vi "Periodic Tasks.vi"(8 "error in":errorcluster) -> ()   [LabVIEW 2016]
doc: "This VI runs in parallel to other tasks. It can contain as many user-defined periodic loops as you need. These can carry out PID or other sorts of timed response."
uses:
  MotionProfileClass/MotionProfiles.lvclass
  <vilib>/Rock Robotics/WPI/ThirdParty/CanMotor/TalonSRX/WPI_CANTalonSRX_APIControlMode.ctl
  <vilib>/Rock Robotics/WPI/Utilities/WPI_GetSetVariantRefNum.vi
panel:
  out "Left Prof Count":i32
  out "Right Prof Count":i32
  out "Right Throttle":dbl(graph)
  out "Right Motor":T1(graph)
  out "Left Throttle":dbl(graph)
  out "Left Motor":T1(graph)
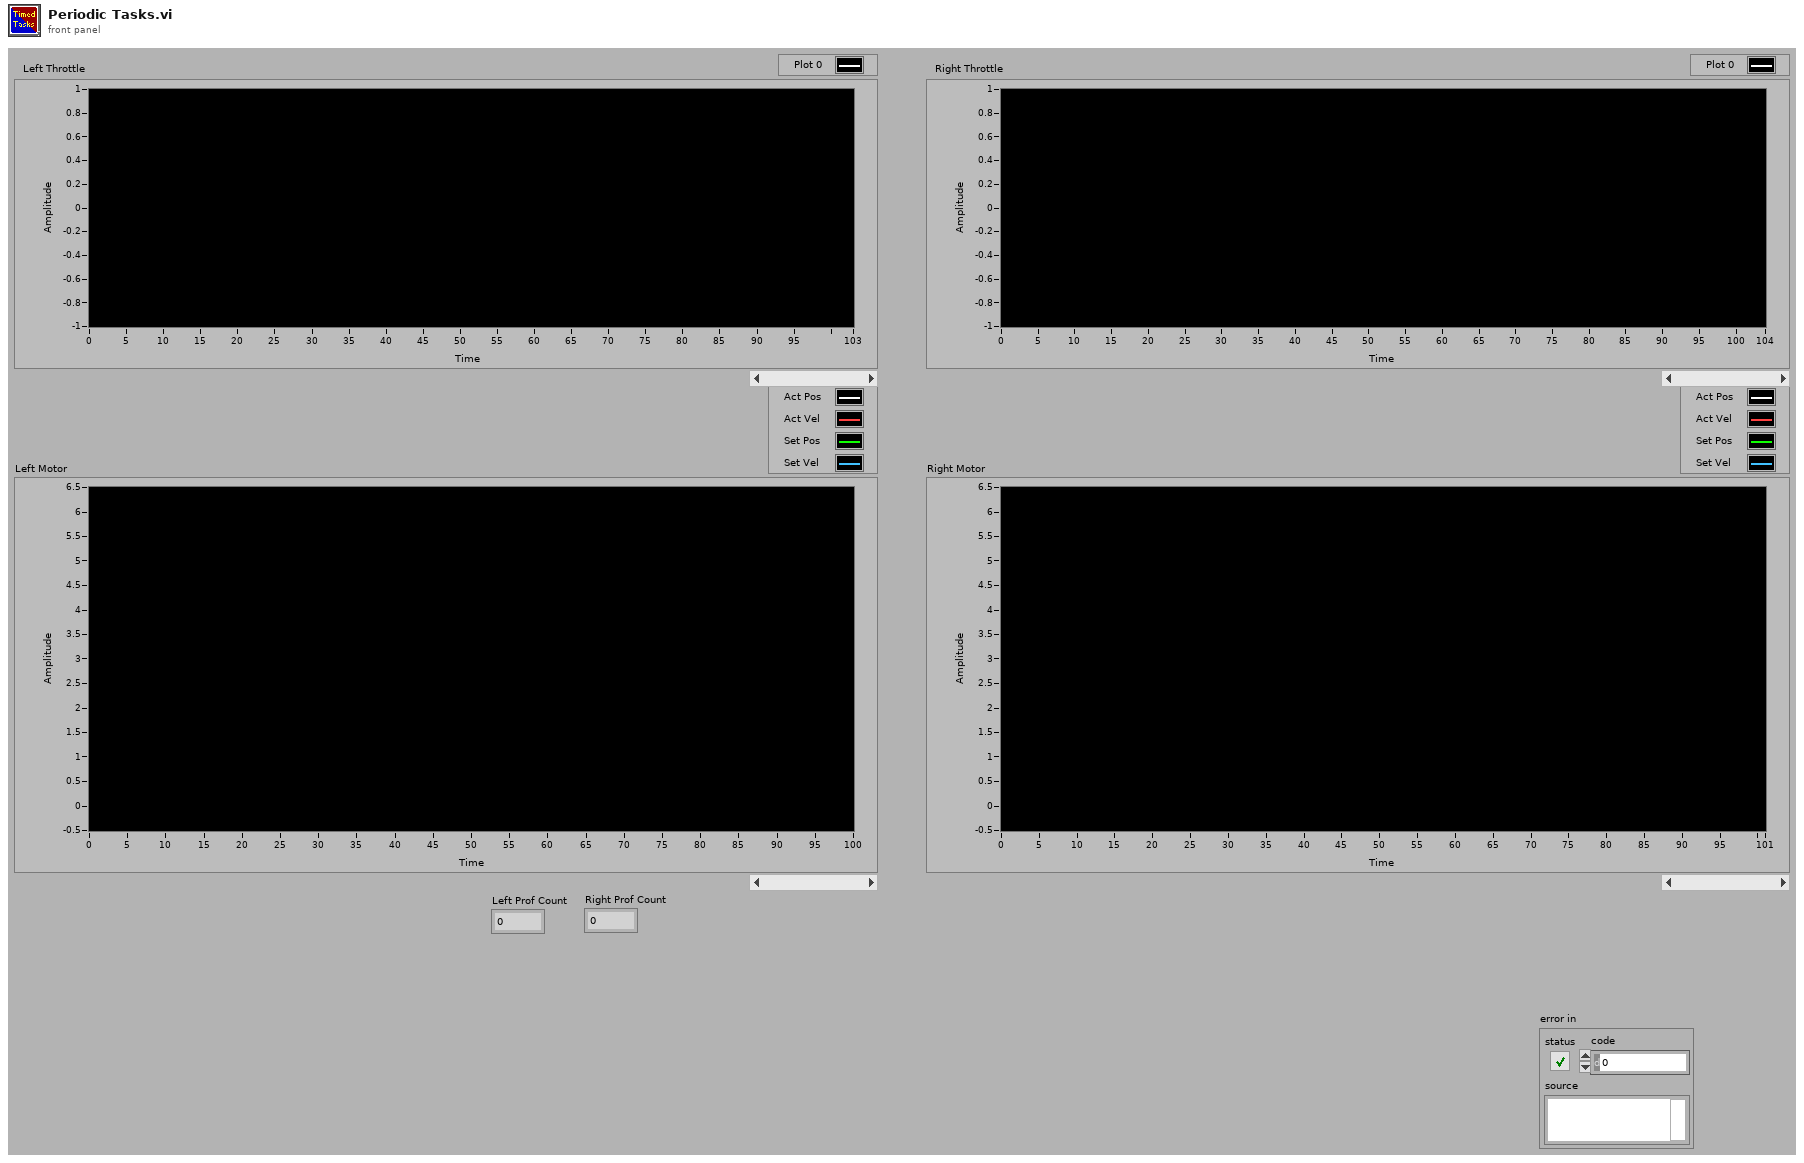
[diagram p1: front panel]
types:
  T1 = cluster{"Sensor Position":dbl, "Sensor Velocity":dbl, "Mot Prof Active Position":dbl, "Mot Prof Active Velocity":dbl}
  T2 = typedef "WPI_MotorControlDeviceRef.ctl" = cluster{"DeviceStatus":errorcluster, "Type":T3, "PWM":cluster{"PWM Channel":T4, "DeadBand":T5}, "CAN":cluster{"Device Number":u8, "SetOutput VI Ref":variant, "GetOutput VI Ref":variant, "Enable VI Ref":variant, "Disable VI Ref":variant, "Data":variant}, "Invert":bool}
  T3 = typedef "WPI_MotorControlType.ctl" = enum16{"PWM", "CAN"}
  T4 = typedef "FPGA_DIOPWMChannel.ctl" = enum8{"PWM 0", "PWM 1", "PWM 2", "PWM 3", "PWM 4", "PWM 5", "PWM 6", "PWM 7", "PWM 8", "PWM 9", "PWM MXP 0", "PWM MXP 1", "PWM MXP 2", "PWM MXP 3", "PWM MXP 4", "PWM MXP 5", "PWM MXP 6", "PWM MXP 7", "PWM MXP 8", "PWM MXP 9", "Invalid"}
  T5 = typedef "WPI_PWMDeadband.ctl" = cluster{"Name":string, "maxPositivePwm":i32, "minPositivePwm":i32, "centerPwm":i32, "maxNegativePwm":i32, "minNegativePwm":i32, "angularRange":u16}
  T6 = typedef "WPI_JoystickDevRef.ctl" = cluster{"Device":T7}
  T7 = typedef "WPI_JoystickDeviceEnum.ctl" = enum16{"USB 0", "USB 1", "USB 2", "USB 3", "USB 4", "USB 5"}
  T8 = typedef "WPI_CANTalonSRX_APIControlMode.ctl" = enum8{"Percent VBus", "Speed", "Position", "Slave", "Unchanged / Invalid", "Voltage Compensation", "Current", "Motion Profile", "Motion Magic"}
  T9 = typedef "MotionProfiles.lvclass/MotionProfile_TalonSetValueEnum.ctl" = enum16{"Disable", "Enable", "Hold"}
  T10 = typedef "WPI_CANTalonSRX_GlobalStatus.ctl" = cluster{"Applied Throttle":dbl, "Module Enabled":bool, "CAN Error":errorcluster, "Closed Loop Error":dbl, "Forward Limit Switch Closed":bool, "Reverse Limit Switch Closed":bool, "Sensor Position":dbl, "Sensor Velocity":dbl, "Current":dbl, "Sticky Fault - Over Temp":bool, "Sticky Fault - Under Voltage":bool, "Sticky Fault - Forward Limit":bool, "Sticky Fault - Reverse Limit":bool, "Sticky Fault - Forward Soft Limit":bool, "Sticky Fault - Reverse Soft Limit":bool, "Brake is Enabled":bool, "Encoder Position":dbl, "Encoder Velocity":dbl, "Encoder Index Count":dbl, "Encoder A Pin State":bool, "Encoder B Pin State":bool, "Encoder Index Pin State":bool, "Analog In":dbl, "Analog In Velocity":dbl, "Temperature (C)":dbl, "Battery Voltage":dbl, "Control 5 Is Supported":bool, "Current Profile Slot Select":dbl, "Pos Div 8":bool, "Vel Div 4":bool, "Pulse Width Position":i32, "Pulse Width Velocity":i32, "Pulse Width Rise To Rise (us)":i32, "Pulse Width Rise To Fall (us)":i32, "Mot Prof Active Is Under Run":bool, "Mot Prof Active Has Under Run":bool, "Mot Prof Active Is Last":bool, "Mot Prof Active Velocity Only":bool, "Mot Prof Active Is Valid":bool, "Mot Prof Buffer Is Full":bool, "Mot Prof Active Profile Slot Select":i32, "Mot Prof NextID":i32, "Mot Prof Count":i32, "Mot Prof Active Velocity":dbl, "Mot Prof Active Position":dbl, "Mot Prof Output Enable":i32, "UsageFrame":u32, "Motion Magic Active Trajectory":cluster{"Velocity":dbl, "Position":dbl}}
  T11 = cluster{"Sensor Position":dbl, dbl, "Mot Prof Active Position":dbl, dbl}
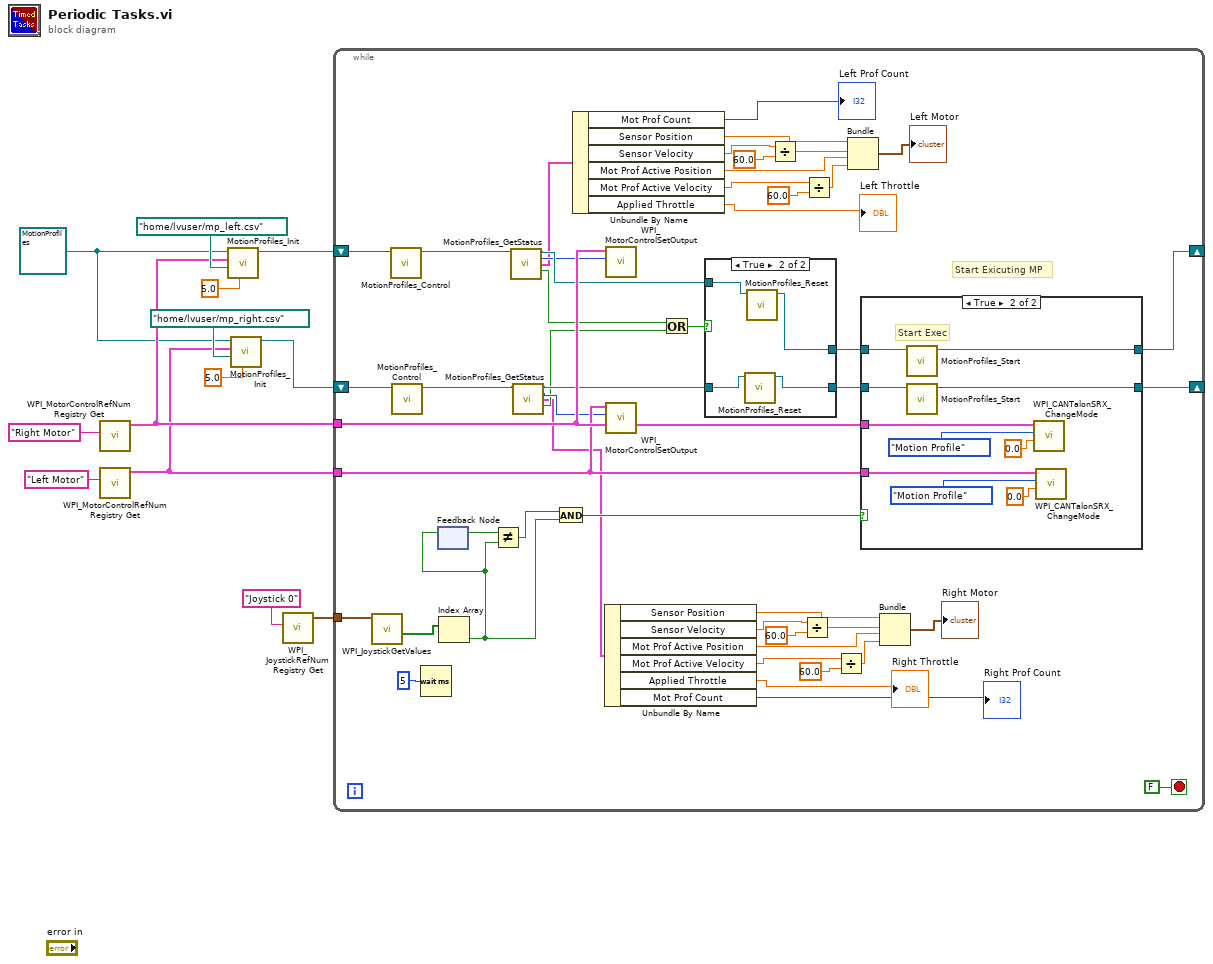
[diagram p0: block diagram]
diagram:
  w1 = refnum<class "MotionProfiles.lvclass"> refnum ("MotionProfiles.lvclass")
  n1 = call <vilib>:"WPI_MotorControlRefNum Registry Get.vi"("refnum name"="Right Motor") -> ("MotorControlDevRef"=w8:T2)  [unwired: 9 in, 1 out]
  n2 = call <vilib>:"WPI_MotorControlRefNum Registry Get.vi"("refnum name"="Left Motor") -> ("MotorControlDevRef"=w2:T2)  [unwired: 9 in, 1 out]
  n3 = call "MotionProfiles_Init.vi"("MP Frame Rate"=5.0, "CSV File Path"=path "/home/lvuser/mp_left.csv" ("file path (use dialog)"), "CAN Talon SRX Ref"=w8, "MotionProfiles in"=w1) -> ("MotionProfiles out"=w10:refnum<class "MotionProfiles.lvclass">)  [unwired: 5 in, 1 out]
  n4 = call "MotionProfiles_Init.vi"("MP Frame Rate"=5.0, "CSV File Path"=path "/home/lvuser/mp_right.csv" ("file path (use dialog)"), "CAN Talon SRX Ref"=w2, "MotionProfiles in"=w1) -> ("MotionProfiles out"=w3:refnum<class "MotionProfiles.lvclass">)  [unwired: 5 in, 1 out]
  n5 = call <vilib>:"WPI_JoystickRefNum Registry Get.vi"("refnum name"="Joystick 0") -> ("JoystickDevRef"=w7:T6)  [unwired: 1 in, 9 out]
  n6 = while {
    tunnel: w8 -> [w54]
    tunnel: w7 -> [w59]
    tunnel: w2 -> [w53]
    shift-right: [w51] -> _
    shift-left: w10 -> [w60]
    shift-right: [w52] -> _
    shift-left: w3 -> [w57]
    stop <- FALSE stop-if-true
    # "Start Exicuting MP"
    n7 = call <vilib>:"WPI_JoystickGetValues.vi"("JoystickDevRef"=w59) -> ("Buttons"=w58:bool[])  [unwired: 6 in, 4 out]
    n8 = call "MotionProfiles_Control.vi"("MotionProfiles in"=w60) -> ("MotionProfiles out"=w45:refnum<class "MotionProfiles.lvclass">)  [unwired: 9 in, 1 out]
    n9 = call "MotionProfiles_Control.vi"("MotionProfiles in"=w57) -> ("MotionProfiles out"=w41:refnum<class "MotionProfiles.lvclass">)  [unwired: 9 in, 1 out]
    n10 = Wait (ms)(milliseconds to wait=u32 5) -> ()  [unwired: 1 out]
    n11 = feedback #1() -> (w47:bool)  [unwired: 1 in]
    n12 = Index Array(array=w58) -> (element=w46:bool)  [unwired: 1 in]
    n13 = feedback-in #1(w46) -> ()
    n14 = Not Equal?(x=w47, y=w46) -> (x != y?=w56:bool)
    n15 = call "MotionProfiles_GetStatus.vi"("MotionProfiles in"=w45) -> ("MotionProfiles out"=w44:refnum<class "MotionProfiles.lvclass">, "TalonSetValue"=w43:T9, "Talon SRX Status"=w37:T10, "MP Is Done"=w42:bool)  [unwired: 10 in, 1 out]
    n16 = call "MotionProfiles_GetStatus.vi"("MotionProfiles in"=w41) -> ("MotionProfiles out"=w40:refnum<class "MotionProfiles.lvclass">, "TalonSetValue"=w39:T9, "Talon SRX Status"=w16:T10, "MP Is Done"=w38:bool)  [unwired: 10 in, 1 out]
    n17 = And(x=w56, y=w46) -> (x .and. y?=w55:bool)
    n18 = Unbundle By Name(w37) -> ("Mot Prof Count"=→"Left Prof Count":i32, "Sensor Position"=w36:dbl, "Sensor Velocity"=w27:dbl, "Mot Prof Active Position"=w30:dbl, "Mot Prof Active Velocity"=w32:dbl, "Applied Throttle"=→"Left Throttle":dbl)
    n19 = Unbundle By Name(w16) -> ("Sensor Position"=w26:dbl, "Sensor Velocity"=w17:dbl, "Mot Prof Active Position"=w20:dbl, "Mot Prof Active Velocity"=w22:dbl, "Applied Throttle"=→"Right Throttle":dbl, "Mot Prof Count"=→"Right Prof Count":i32)
    n20 = call <vilib>:"WPI_MotorControlSetOutput.vi"("Output"=w43, "MotorControlDevRef"=w54) -> ()  [unwired: 7 in, 3 out]
    n21 = call <vilib>:"WPI_MotorControlSetOutput.vi"("Output"=w39, "MotorControlDevRef"=w53) -> ()  [unwired: 7 in, 3 out]
    n22 = Or(x=w42, y=w38) -> (x .or. y?=w48:bool)
    n23 = case shown="True" w48 {
      tunnel: w44 -> [w64 w68]
      tunnel: [w64 w67] -> w50
      tunnel: w40 -> [w63 w66]
      tunnel: [w63 w65] -> w49
      frame False {
      }
      frame True {
        n24 = call "MotionProfiles_Reset.vi"("MotionProfiles in"=w66) -> ("MotionProfiles out"=w65:refnum<class "MotionProfiles.lvclass">)  [unwired: 9 in, 1 out]
        n25 = call "MotionProfiles_Reset.vi"("MotionProfiles in"=w68) -> ("MotionProfiles out"=w67:refnum<class "MotionProfiles.lvclass">)  [unwired: 9 in, 1 out]
      }
    }
    n26 = Divide(x=w27, y=60.0) -> (x/y=w28:dbl)
    n27 = Divide(x=w17, y=60.0) -> (x/y=w18:dbl)
    n28 = Divide(x=w32, y=60.0) -> (x/y=w33:dbl)
    n29 = Divide(x=w22, y=60.0) -> (x/y=w23:dbl)
    n30 = Bundle("Sensor Position"=w36, w28, "Mot Prof Active Position"=w30, w33) -> (→"Left Motor":T11)  [unwired: 1 in]
    n31 = case shown="True" w55 {
      tunnel: w50 -> [w70 w80]
      tunnel: w54 -> [_ w79]
      tunnel: w49 -> [w69 w77]
      tunnel: w53 -> [_ w74]
      tunnel: [w69 w72] -> w52
      tunnel: [w70 w71] -> w51
      frame False {
      }
      frame True {
        # "Start Exec"
        n32 = call "MotionProfiles_Start.vi"("MotionProfiles in"=w80) -> ("MotionProfiles out"=w71:refnum<class "MotionProfiles.lvclass">)  [unwired: 9 in, 1 out]
        n33 = call "MotionProfiles_Start.vi"("MotionProfiles in"=w77) -> ("MotionProfiles out"=w72:refnum<class "MotionProfiles.lvclass">)  [unwired: 9 in, 1 out]
        n34 = call <vilib>:"WPI_CANTalonSRX_ChangeMode.vi"("Output"=0.0, "Control Mode"=WPI_CANTalonSRX_APIControlMode."Motion Profile", "CAN Talon SRX Ref"=w79) -> ()  [unwired: 7 in, 2 out]
        n35 = call <vilib>:"WPI_CANTalonSRX_ChangeMode.vi"("Output"=0.0, "Control Mode"=WPI_CANTalonSRX_APIControlMode."Motion Profile", "CAN Talon SRX Ref"=w74) -> ()  [unwired: 7 in, 2 out]
      }
    }
    n36 = Bundle("Sensor Position"=w26, w18, "Mot Prof Active Position"=w20, w23) -> (→"Right Motor":T11)  [unwired: 1 in]
  }
